vi "Read MAG.vi"(8 "error in (no error)":errorcluster, 11 "Referential in":refnum<class "Referential.lvclass">) -> (0 "error out":errorcluster, 2 "MAG":dbl, 3 "Referential out":refnum<class "Referential.lvclass">)   [LabVIEW 2019, in "Referential.lvclass"]
uses:
  Referential.lvclass
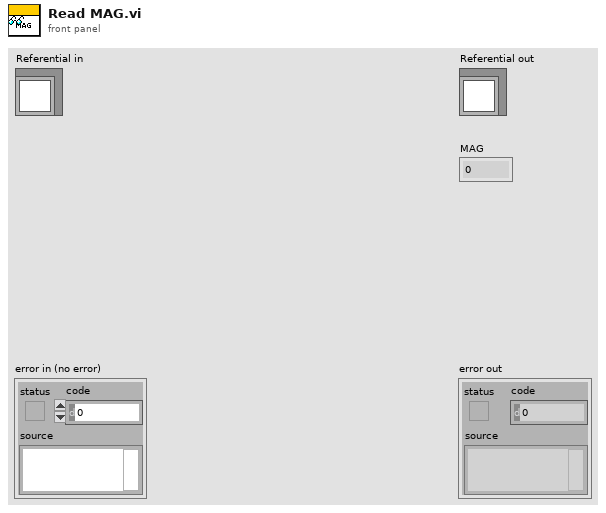
[diagram p1: front panel]
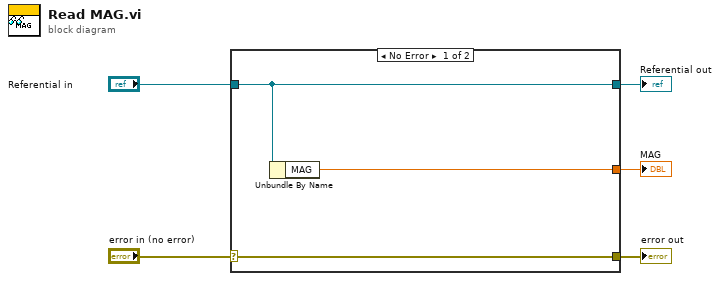
[diagram p0: block diagram]
diagram:
  n1 = case shown="No Error" "error in (no error)" {
    selector: "error in (no error)" -> [w8 w9]
    tunnel: [w8 w9] -> w4
    tunnel: [w7 w10] -> w2
    tunnel: "Referential in" -> [w7 w10]
    tunnel: [w6 _] -> w1
    frame No Error {
      n2 = Unbundle By Name(w7) -> ("MAG"=w6:dbl)
    }
    frame Error {
    }
  }
  "error out" <- w4
  "Referential out" <- w2
  "MAG" <- w1
